vi "ConnectionHeaderReply.vi"(2 "type":string, 3 "Latching":string, 4 "Caller ID":string, 5 "TCPROS Connection Header":string) -> (1 "Connection Response":string)   [LabVIEW 2014]
doc: "Returns the connection response from the connection header"
uses:
  <userlib>/ROS for LabVIEW Software.lnk/ROS/MessageBuilding/std_msgs/subs/stringArray.vi
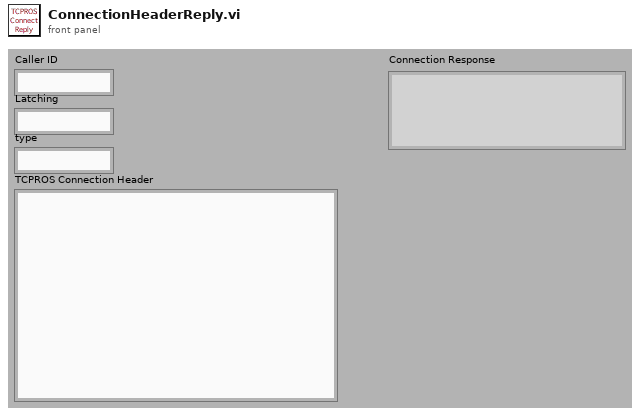
[diagram p1: front panel]
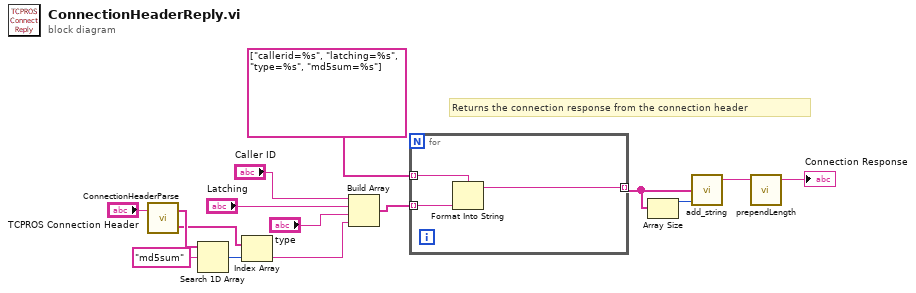
[diagram p0: block diagram]
diagram:
  # "Returns the connection response from the connection header"
  n1 = call <userlib>:"ConnectionHeaderParse.vi"("TCPROS Connection Header"="TCPROS Connection Header") -> ("Values"=w8:string[], "Fields"=w10:string[])  [unwired: 1 in]
  n2 = Search 1D Array(1D array=w10, element="md5sum") -> (index of element=w7:i32)  [unwired: 1 in]
  n3 = Index Array(array=w8, index=w7) -> (element=w6:string)
  n4 = Build Array("Caller ID", "Latching", "type", w6) -> (w14:string[])
  n5 = for {
    tunnel: string[] ["callerid=%s", "latching=%s", "type=%s", "md5sum=%s"] -> [w18] mode=indexing
    tunnel: w14 -> [w17] mode=indexing
    tunnel: [w16] -> w2 mode=indexing
    n6 = Format Into String(format string=w18, w17) -> (resulting string=w16:string)  [unwired: 2 in, 1 out]
  }
  n7 = Array Size(array=w2) -> (size(s)=w1:i32)
  n8 = call-poly <userlib>:"add_string.vi"("Array Length"=w1, "Array"=w2) -> ("msg out"=w4:string)  [unwired: 3 in]
  n9 = call <userlib>:"prependLength.vi"("msg in"=w4) -> ("msg out"=→"Connection Response":string)  [unwired: 4 in]
